vi "S2C_Shared_Proc_SendLocalCmd.vi"(8 "Error In":errorcluster, 9 "ExeRef":refnum<vi>, 11 "Q-Ref":refnum<queue>) -> (0 "Error Out":errorcluster, 3 "Command":string)   [LabVIEW 2024]
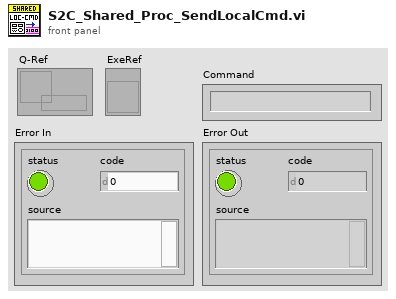
[diagram p1: front panel]
types:
  T1 = cluster{"Caller-Q":refnum<queue>, "Command":string, "Return":string, "Data":variant, "Timeout":dbl}
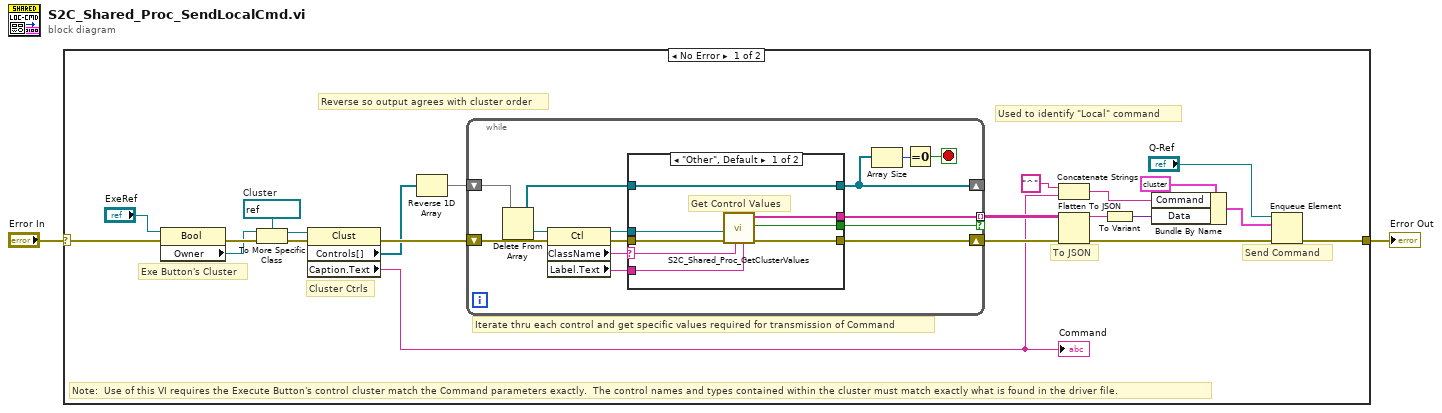
[diagram p0: block diagram]
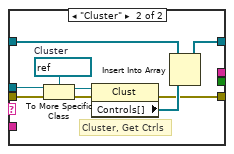
[diagram p2: hidden frame]
diagram:
  n1 = case shown="No Error" "Error In" {
    selector: "Error In" -> [w23 w56]
    tunnel: [w4 w56] -> w1
    frame No Error {
      w20 = refnum<vi> refnum  # Cluster
      # "Reverse so output agrees with cluster order"
      # "Note:  Use of this VI requires the Execute Button's control cluster match the Command parameters exactly.  The control names and types contained within the cluster must match exactly what is found in the driver file."
      # "Used to identify \"Local\" command"
      # "Send Command"
      # "To JSON"
      # "Iterate thru each control and get specific values required for transmission of Command"
      # "Cluster Ctrls"
      # "Exe Button's Cluster"
      n2 = property class="Bool"(reference="ExeRef", error in=w23) -> (error out=w22:errorcluster, "Owner"=w21:refnum<vi>)  [unwired: 1 out]
      n3 = To More Specific Class(target class=w20, reference=w21, error in=w22) -> (specific class reference=w18:refnum<vi>, error out=w19:errorcluster)
      n4 = property class="Clust"(reference=w18, error in=w19) -> (error out=w17:errorcluster, "Controls[]"=w6:refnum<vi>[], "Caption.Text"=w3:string)  [unwired: 1 out]
      "Command" <- w3
      n5 = Reverse 1D Array(array=w6) -> (reversed array=w5:refnum<vi>[])
      n6 = while {
        shift-right: [w32] -> _
        shift-left: w5 -> [w38]
        shift-right: [w29] -> w8
        shift-left: w17 -> [w37]
        tunnel: [w27] -> w7 mode=indexing if=w26
        stop <- w30 stop-if-true
        n7 = Delete From Array(array=w38) -> (deleted portion=w36:refnum<vi>, array with subset deleted=w33:refnum<vi>[])  [unwired: 2 in]
        n8 = property class="Ctl"(reference=w36, error in=w37) -> (reference out=w28:refnum<vi>, error out=w35:errorcluster, "ClassName"=w34:string, "Label.Text"=w25:string)
        n9 = case shown="\"Other\", Default" w34 {
          selector: w34 -> [w44 _]
          tunnel: w35 -> [w46 w51]
          tunnel: w33 -> [w42 w50]
          tunnel: [w42 w49] -> w32
          tunnel: [w43 w48] -> w29
          tunnel: w28 -> [w45 w47]
          tunnel: [w41 _] -> w27
          tunnel: [w40 _] -> w26
          tunnel: w25 -> [w39 _]
          frame "Other", Default {
            # "Get Control Values"
            n10 = call "S2C_Shared_Proc_GetClusterValues.vi"("LabelText"=w39, "ClassName"=w44, "Error In"=w46, "CtrlRef"=w45) -> ("Error Out"=w43:errorcluster, "Valid?"=w40:bool, "Settings"=w41:string[])  [unwired: 5 in]
          }
          frame "Cluster" {
            w55 = refnum<vi> refnum  # Cluster
            # "Cluster, Get Ctrls"
            n11 = To More Specific Class(target class=w55, reference=w47, error in=w51) -> (specific class reference=w53:refnum<vi>, error out=w54:errorcluster)
            n12 = property class="Clust"(reference=w53, error in=w54) -> (error out=w48:errorcluster, "Controls[]"=w52:refnum<vi>[])  [unwired: 1 out]
            n13 = Insert Into Array(array=w50, new element=w52) -> (w49:refnum<vi>[])  [unwired: 1 in]
          }
        }
        n14 = Array Size(array=w32) -> (size(s)=w31:i32)
        n15 = Equal To 0?(x=w31) -> (x = 0?=w30:bool)
      }
      n16 = Concatenate Strings("^" ("string"), w3) -> (w9:string)
      n17 = Flatten To JSON(anything=w7, error in (no error)=w8) -> (JSON string=w11:string, 11:w16:errorcluster)  [unwired: 1 in]
      n18 = To Variant(anything=w11) -> (Variant=w13:variant)
      n19 = Bundle By Name(cluster=T1 {"Caller-Q"=refnum, "Command"="", "Return"="None", "Data"=variant, "Timeout"=10.0} ("element"), "Command"=w9, "Data"=w13) -> (w12:T1)
      n20 = Enqueue Element(queue="Q-Ref", element=w12, error in (no error)=w16) -> (error out=w4:errorcluster)  [unwired: 1 in, 2 out]
    }
    frame Error {
    }
  }
  "Error Out" <- w1
